vi "Validate Application_Name.vi"(8 "Error In":errorcluster, 11 "Application_Name":string) -> (0 "Error Out":errorcluster)   [LabVIEW 2023, in "Error Manager.lvlib" / "Settings.lvclass"]
doc: "This VI performs one or more validation checks on the <B>Application_Name</B> setting value read from file.\n\nError Behaviour\n1. The VI skips execution if \"Error In\" contains an error. The input error is passed-through unaltered.\n2. If all validation checks passed the VI outputs \"No Error\".\n3. If a validation check failed the VI outputs an error with an informative error message."
uses:
  Settings.lvclass
  Settings.lvclass/Settings.ctl
  Error Manager.lvlib
  <vilib>/Utility/error.llb/whitespace.ctl
panel:
  # "Development\nControls or indicators that are useful for development or testing, but which are not outputs of the VI."
  # "Input\nInputs to the VI"
  # "Output\nOutputs of the VI"
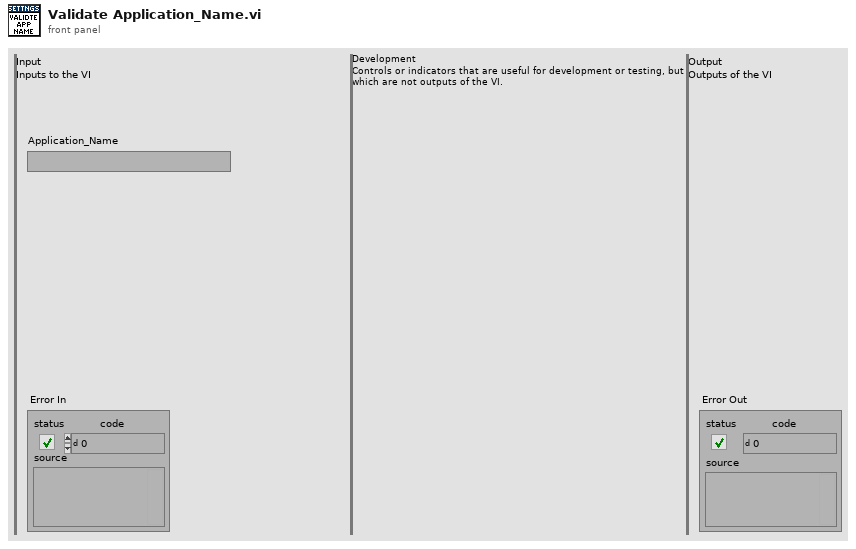
[diagram p1: front panel]
types:
  T1 = typedef "whitespace.ctl" = u16
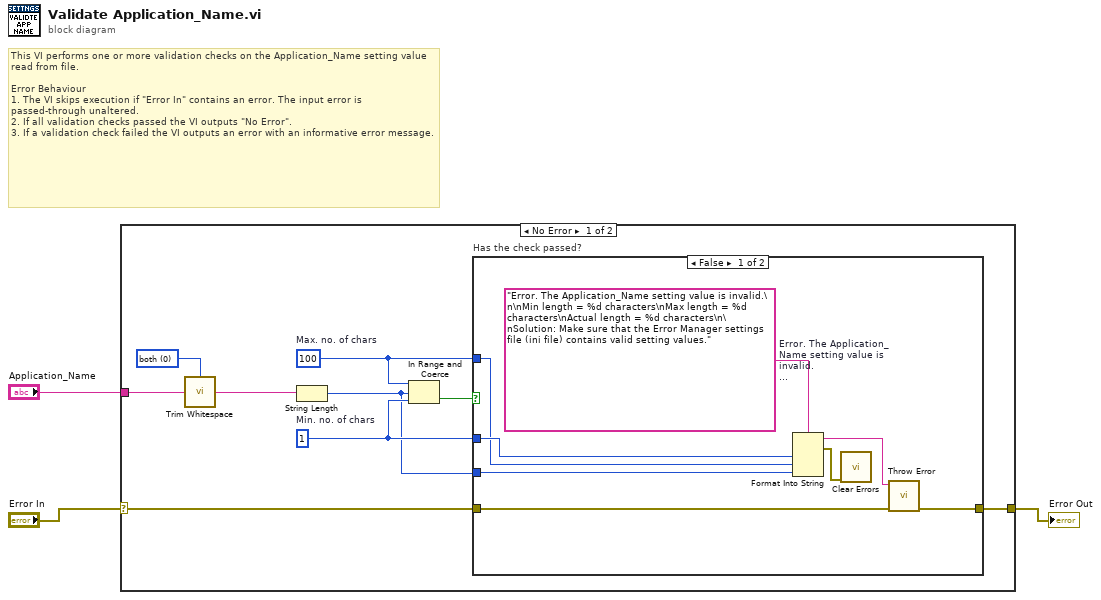
[diagram p0: block diagram]
diagram:
  # "This VI performs one or more validation checks on the Application_Name setting value read from file.\n\nError Behaviour\n1. The VI skips execution if \"Error In\" contains an error. The input error is passed-through unaltered.\n2. If all validation checks passed the VI outputs \"No Error\".\n3. If a validation check failed the VI outputs an error with an informative error message."
  n1 = case shown="No Error" "Error In" {
    selector: "Error In" -> [w12 w22]
    tunnel: [w10 w22] -> w2
    tunnel: "Application_Name" -> [w11 _]
    frame No Error {
      w4 = T1 0 items=["both", "start of string", "end of string"] ("location (both)")
      w7 = 100  # Max. no. of chars
      w8 = 1  # Min. no. of chars
      n2 = call <vilib>:"Trim Whitespace.vi"("string"=w11, "location (both)"=w4) -> ("trimmed string"=w5:string)
      n3 = String Length(string=w5) -> (length=w6:i32)
      n4 = In Range and Coerce(upper limit=w7, x=w6, lower limit=w8) -> (In Range?=w9:bool)  [unwired: 1 out]
      n5 = case "Has the check passed?" shown="False" w9 {
        tunnel: w12 -> [w20 w21]
        tunnel: [w19 w21] -> w10
        tunnel: w8 -> [w15 _]
        tunnel: w7 -> [w14 _]
        tunnel: w6 -> [w13 _]
        frame False {
          w16 = "Error. The Application_Name setting value is invalid.\n\nMin length = %d characters\nMax length = %d characters\nActual length = %d characters\n\nSolution: Make sure that the Error Manager settings file (ini file) contains valid setting values."  # Error. The Application_Name setting value is invalid.  Min length = %d characters Max length = %d characters Actual length = %d characters  Solution: Make sure that the Error Manager settings file (ini file) contains valid setting values.
          n6 = Format Into String(format string=w16, w15, w14, w13) -> (resulting string=w17:string, error out=w18:errorcluster)  [unwired: 2 in]
          n7 = call <vilib>:"Clear Errors.vi"("error in (no error)"=w18) -> ()  [unwired: 5 in, 2 out]
          n8 = call "Throw Error.vi"("error in"=w20, "Error Message"=w17) -> ("error out"=w19:errorcluster)  [unwired: 9 in]
        }
        frame True {
        }
      }
    }
    frame Error {
    }
  }
  "Error Out" <- w2
